vi "2021 Advent puzzle 05 Handle inp line.vi"(10 "String":string="0,9 -> 5,9") -> (0 "error out":errorcluster, 1 "y2":i32, 2 "x2":i32, 3 "y1":i32, 5 "x1":i32)   [LabVIEW 2021]
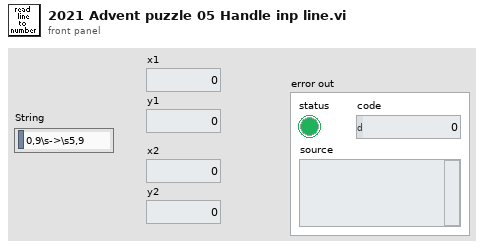
[diagram p1: front panel]
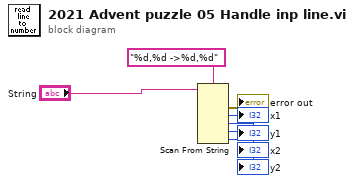
[diagram p0: block diagram]
diagram:
  n1 = Scan From String(format string="%d,%d ->%d,%d", input string="String") -> (error out=→"error out":errorcluster, output 1=→"x1":i32, output 2=→"y1":i32, output 3=→"x2":i32, output 4=→"y2":i32)  [unwired: 6 in, 2 out]
